vi "Configure_PSG_ Frequency_Power_final.vi"(1 "Attenuator Auto Mode (T:Enable)":bool=TRUE, 2 "Power [dBm]":dbl=-130.0, 3 "Frequency [GHz]":dbl=100000.0) -> ()   [LabVIEW 2011]
doc: "This example shows how to configure the frequency and power of the output signal."
uses:
  <vilib>/Utility/error.llb/DialogType.ctl
  <instrlib>/Agilent PSG MXG Series/Agilent PSG MXG Series.lvlib
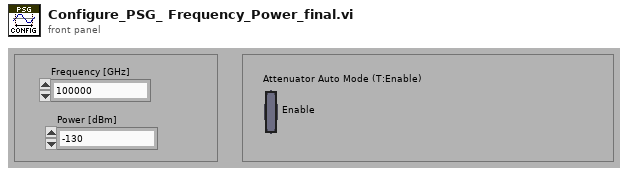
[diagram p1: front panel]
types:
  T1 = typedef "DialogType.ctl" = u16
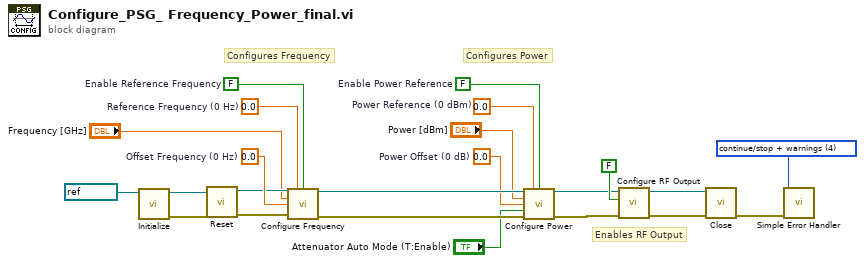
[diagram p0: block diagram]
diagram:
  w2 = T1 4 items=["no dialog", "OK message", "continue or stop message", "OK message + warnings", "continue/stop + warnings"] ("type of dialog (OK msg:1)")
  w14 = 0.0  # Offset Frequency (0 Hz)
  w15 = 0.0  # Reference Frequency (0 Hz)
  w12 = 0.0  # Power Reference (0 dBm)
  w11 = 0.0  # Power Offset (0 dB)
  w13 = FALSE  # Enable Power Reference
  w16 = FALSE  # Enable Reference Frequency
  # "Enables RF Output"
  # "Configures Power"
  # "Configures Frequency"
  n1 = call <instrlib>:"Initialize.vi"("VISA resource name"=refnum<visa-resource-name> "PSG1") -> ("error out"=w4:errorcluster, "VISA resource name out"=w6:refnum<visa-resource-name>)  [unwired: 9 in]
  n2 = call <instrlib>:"Reset.vi"("error in (no error)"=w4, "VISA resource name"=w6) -> ("error out"=w3:errorcluster, "VISA resource name out"=w5:refnum<visa-resource-name>)  [unwired: 8 in]
  n3 = call <instrlib>:"Configure Frequency.vi"("VISA resource name"=w5, "Reference Frequency (0 Hz)"=w15, "Enable Reference Frequency (F:Disable)"=w16, "Frequency (100 kHz)"="Frequency [GHz]", "Offset Frequency (0 Hz)"=w14, "error in (no error)"=w3) -> ("VISA resource name out"=w23:refnum<visa-resource-name>, "error out"=w22:errorcluster)  [unwired: 8 in]
  n4 = call <instrlib>:"Configure Power.vi"("VISA resource name"=w23, "Power Reference (0 dBm)"=w12, "Enable Power Reference (F:Disable)"=w13, "Power (-130 dBm)"="Power [dBm]", "Power Offset (0 dB)"=w11, "Attenuator Auto Mode (T:Enable)"="Attenuator Auto Mode (T:Enable)", "error in (no error)"=w22) -> ("VISA resource name out"=w8:refnum<visa-resource-name>, "error out"=w7:errorcluster)  [unwired: 7 in]
  n5 = call <instrlib>:"Configure RF Output.vi"("error in (no error)"=w7, "Enable RF Output (F:Disable)"=FALSE ("RF Output (T:On)"), "VISA resource name"=w8) -> ("error out"=w19:errorcluster, "VISA resource name out"=w20:refnum<visa-resource-name>)  [unwired: 7 in]
  n6 = call <instrlib>:"Close.vi"("error in (no error)"=w19, "VISA resource name"=w20) -> ("error out"=w21:errorcluster)  [unwired: 9 in]
  n7 = call <vilib>:"Simple Error Handler.vi"("type of dialog (OK msg:1)"=w2, "error in (no error)"=w21) -> ()  [unwired: 3 in, 5 out]
